vi "Create.vi"(8 "error in (no error)":errorcluster, 10 "Transfer Groups":refnum<class "Transfer Group.lvclass">[](array[class]), 11 "Buffer Converter type":refnum<class "Buffer Converter.lvclass">) -> (0 "error out":errorcluster, 3 "Buffer Converter out":refnum<class "Buffer Converter.lvclass">)   [LabVIEW 2017, in "DSF Core.lvlib" / "Buffer Converter.lvclass"]
uses:
  Buffer Converter.lvclass
  Transfer Group/Transfer Group.lvclass
  Buffer Converter.lvclass/Buffer Converter.ctl
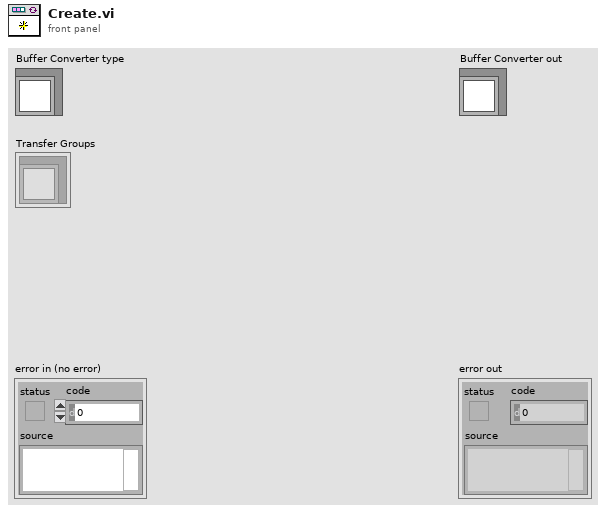
[diagram p1: front panel]
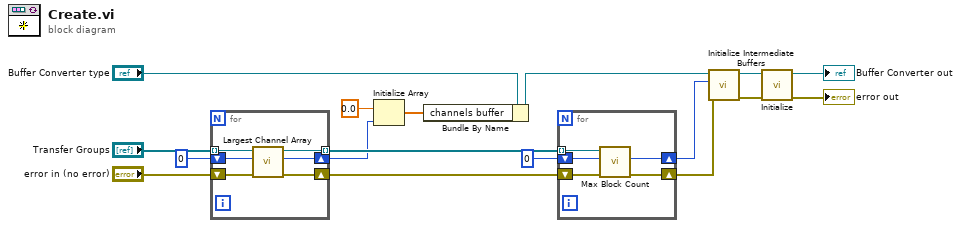
[diagram p0: block diagram]
diagram:
  n1 = for {
    tunnel: "Transfer Groups" -> [w23] mode=indexing
    shift-right: [w19] -> w7
    shift-left: u64 0 ("max channel count") -> [w22]
    shift-right: [w20] -> w15
    shift-left: "error in (no error)" -> [w21]
    tunnel: [w18] -> w13 mode=indexing
    n2 = call "Largest Channel Array.vi"("error in (no error)"=w21, "largest channel array in (0)"=w22, "Transfer Group in"=w23) -> ("error out"=w20:errorcluster, "largest channel array out"=w19:u64, "Transfer Group out"=w18:refnum<class "Transfer Group.lvclass">)  [unwired: 6 in]
  }
  n3 = Initialize Array(0.0 ("element"), w7) -> (w6:dbl[])
  n4 = Bundle By Name(cluster="Buffer Converter type", "channels buffer"=w6) -> (w9:refnum<class "Buffer Converter.lvclass">)
  n5 = for {
    tunnel: w13 -> [w28] mode=indexing
    shift-right: [w24] -> w5
    shift-left: u64 0 ("max channel count") -> [w27]
    shift-right: [w25] -> w11
    shift-left: w15 -> [w26]
    n6 = call "Max Block Count.vi"("error in (no error)"=w26, "previous block count (0)"=w27, "Transfer Group in"=w28) -> ("error out"=w25:errorcluster, "largest block count"=w24:u64)  [unwired: 6 in, 1 out]
  }
  n7 = call "Initialize Intermediate Buffers.vi"("error in (no error)"=w11, "largest block count"=w5, "Buffer Converter in"=w9) -> ("error out"=w1:errorcluster, "Buffer Converter out"=w4:refnum<class "Buffer Converter.lvclass">)  [unwired: 7 in]
  n8 = call-dynamic "Initialize.vi"("error in (no error)"=w1, "Buffer Converter in"=w4) -> ("error out"=→"error out":errorcluster, "Buffer Converter out"=→"Buffer Converter out":refnum<class "Buffer Converter.lvclass">)  [unwired: 8 in]
